vi "imapcgi.vi"   [LabVIEW 2012]
uses:
  <vilib>/addons/internet/NI_InternetTK_Core_VIs.lvlib
types:
  T1 = typedef "CGI Connection Info.ctl" = cluster{"name":string, "type":T2, "session":T3}
  T2 = typedef "CGI Request Type.ctl" = enum16{"cgi", ".spool first", ".spool", ".spool last"}
  T3 = typedef "HTTP Session.ctl" = refnum<k1>
  T4 = typedef "NI_FTP.lvlib/Keyed Array.ctl" = cluster{"keys":string[], "values":string[]}
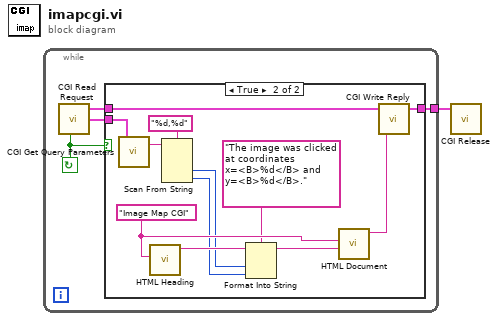
[diagram p0: block diagram]
diagram:
  n1 = while {
    tunnel: [w4] -> w1
    stop <- w3 continue-if-true
    n2 = call <vilib>:"CGI Read Request.vi"() -> ("valid request?"=w3:bool, "cgi connection info"=w5:T1, "env"=w2:T4)  [unwired: 4 in, 1 out]
    n3 = case shown="True" w3 {
      tunnel: [w6 w18] -> w4
      tunnel: w5 -> [w6 w17]
      tunnel: w2 -> [_ w15]
      frame False {
      }
      frame True {
        w14 = "Image Map CGI" ("document title")
        n4 = call <vilib>:"CGI Get Query Parameters.vi"("env"=w15) -> ("query string"=w12:string)  [unwired: 2 out]
        n5 = call <vilib>:"HTML Heading.vi"("heading"=w14) -> ("HTML out"=w10:string)  [unwired: 10 in]
        n6 = Scan From String(format string="%d,%d", input string=w12) -> (output 1=w8:i32, output 2=w7:i32)  [unwired: 4 in, 3 out]
        n7 = Format Into String(format string="The image was clicked at coordinates x=<B>%d</B> and y=<B>%d</B>.", initial string=w10, w8, w7) -> (resulting string=w9:string)  [unwired: 1 in, 1 out]
        n8 = call <vilib>:"HTML Document.vi"("document body"=w9, "document title"=w14) -> ("HTML Document"=w16:string)  [unwired: 9 in]
        n9 = call <vilib>:"CGI Write Reply.vi"("content"=w16, "cgi connection info"=w17) -> ("cgi connection info out"=w18:T1)  [unwired: 3 in]
      }
    }
  }
  n10 = call <vilib>:"CGI Release.vi"("cgi connection info"=w1) -> ()  [unwired: 5 in]
